vi "adjustDACjob.vi"(10 "sample sn":string[](array[string]), 11 "sample port":refnum<visa-resource-name>[](array[refnum])) -> ()   [LabVIEW 2012]
uses:
  globalstatus.vi
  globalsettings.vi
  globalreport.vi
panel:
  out "min":dbl[](array[numeric])
  out "max":dbl[](array[numeric])
  out "real pool":dbl[][](array[numeric])
  in  "times":dbl
  in  "count":dbl
  out "error":errorcluster[](array[cluster])
  in  "blue amp":dbl[](array[numeric])
  in  "red amp":dbl[](array[numeric])
  in  "isred":bool
  out "image":dbl[](array[numeric])
  out "real":dbl[](array[numeric])
  in  "blue dac":dbl[](array[numeric])
  in  "red dac":dbl[](array[numeric])
  in  "Ring":u16(ring) items=["set DAC", "excite", "read"]
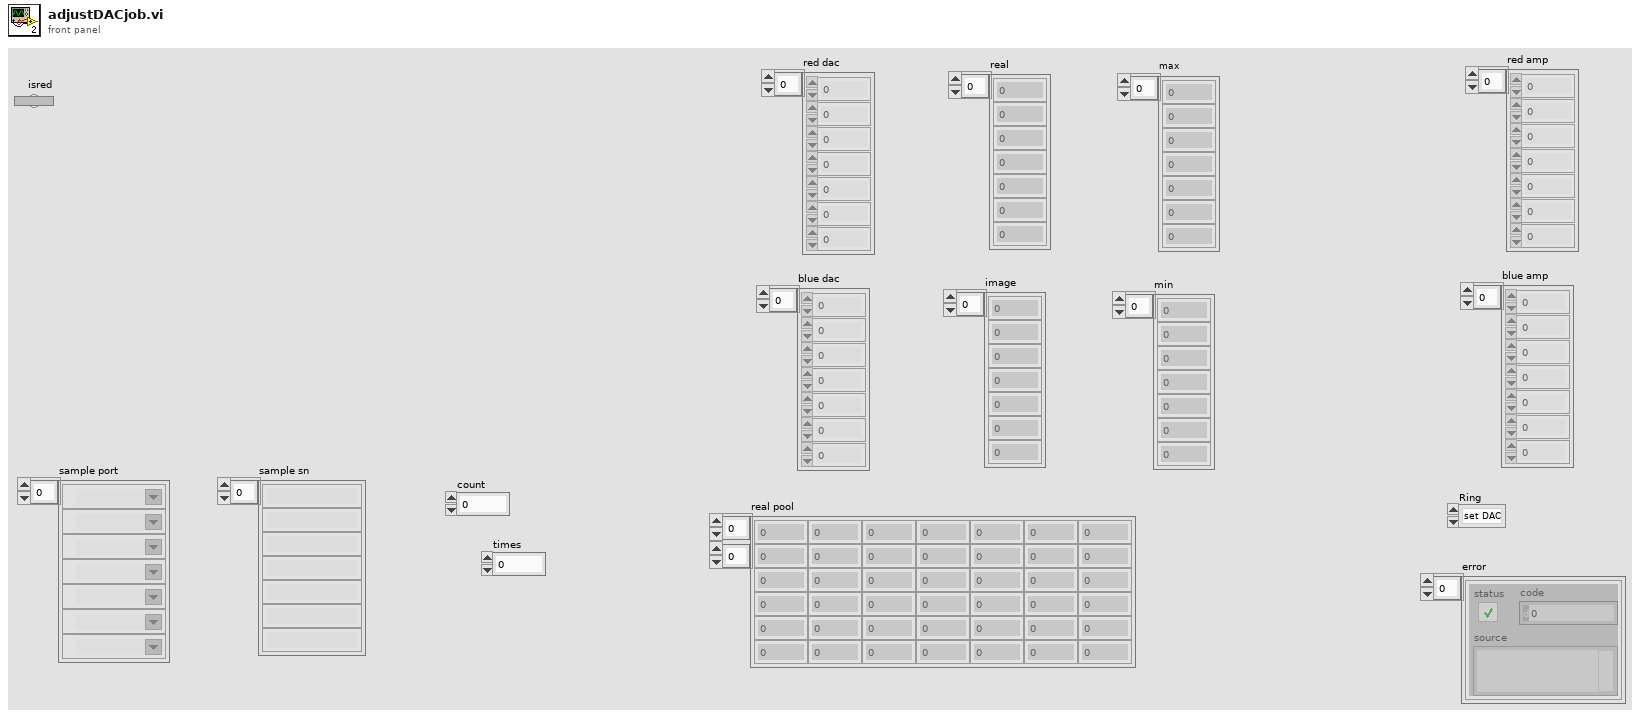
[diagram p1: front panel]
types:
  T1 = cluster{"DAC max":dbl, "DAC min":dbl, "DAC base":dbl, "DAC step":dbl, "Amplitude":dbl, "Tolerance":dbl, "Times":dbl}
  T2 = cluster{"PORT":string, "SN":string, "RED DAC":dbl, "BLUE DAC":dbl, "RED AMP":dbl, "BLUE AMP":dbl, "T0":dbl, "T1":dbl, "T2":dbl, "T3":dbl, "T4":dbl, "T5":dbl, "T6":dbl, "A0":dbl, "A1":dbl, "A2":dbl, "A3":dbl, "B0":dbl, "B1":dbl, "B2":dbl, "C1":dbl, "C0":dbl, "result":string, "error":string}[]
  T3 = cluster{"PORT":string, "SN":string, "RED DAC":dbl, "BLUE DAC":dbl, "RED AMP":dbl, "BLUE AMP":dbl, "T0":dbl, "T1":dbl, "T2":dbl, "T3":dbl, "T4":dbl, "T5":dbl, "T6":dbl, "A0":dbl, "A1":dbl, "A2":dbl, "A3":dbl, "B0":dbl, "B1":dbl, "B2":dbl, "C1":dbl, "C0":dbl, string, string}
  T4 = cluster{"PORT":string, "SN":string, "Numeric":dbl, "Numeric":dbl, "Numeric":dbl, "Numeric":dbl, "T0":dbl, "T1":dbl, "T2":dbl, "T3":dbl, "T4":dbl, "T5":dbl, "T6":dbl, "A0":dbl, "A1":dbl, "A2":dbl, "A3":dbl, "B0":dbl, "B1":dbl, "B2":dbl, "C1":dbl, "C0":dbl, "result":string, "error":string}
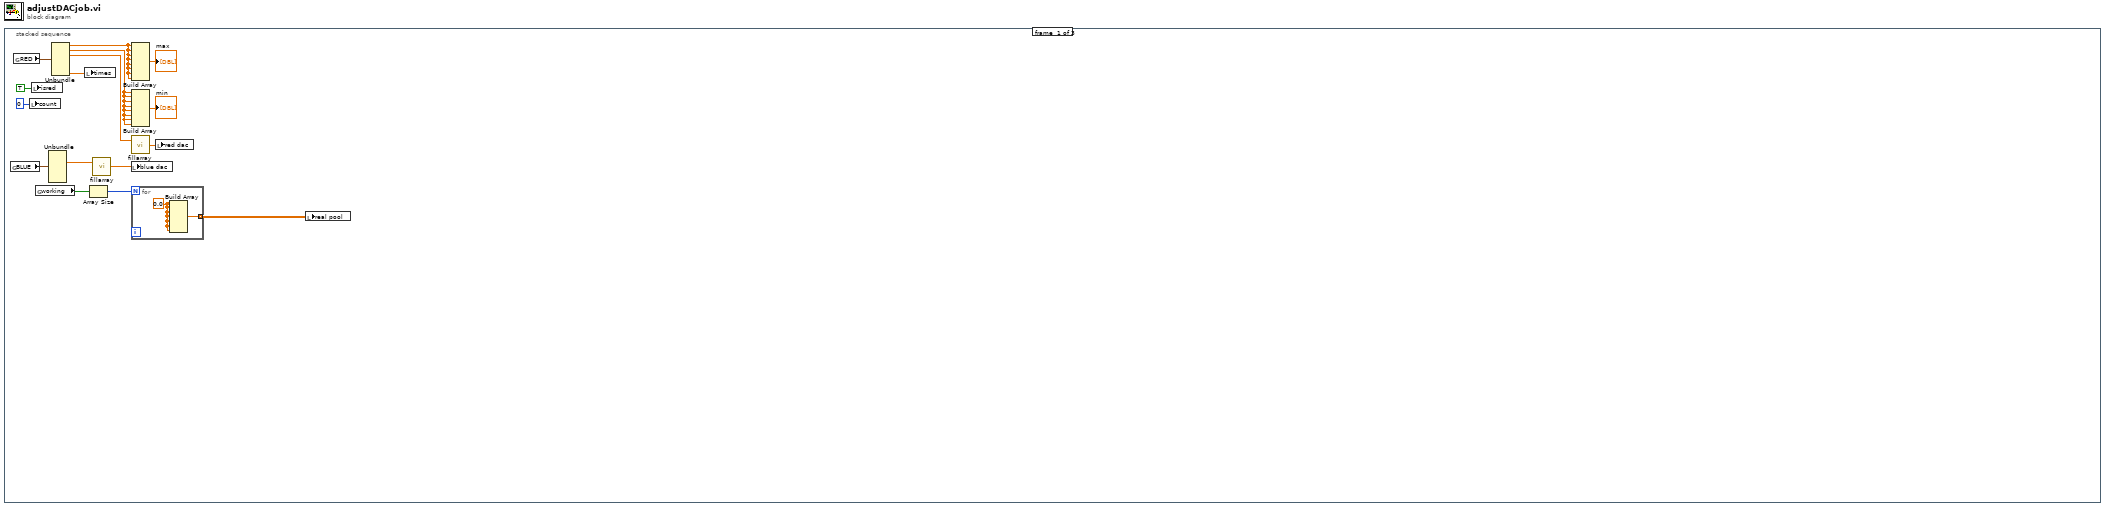
[diagram p0: block diagram]
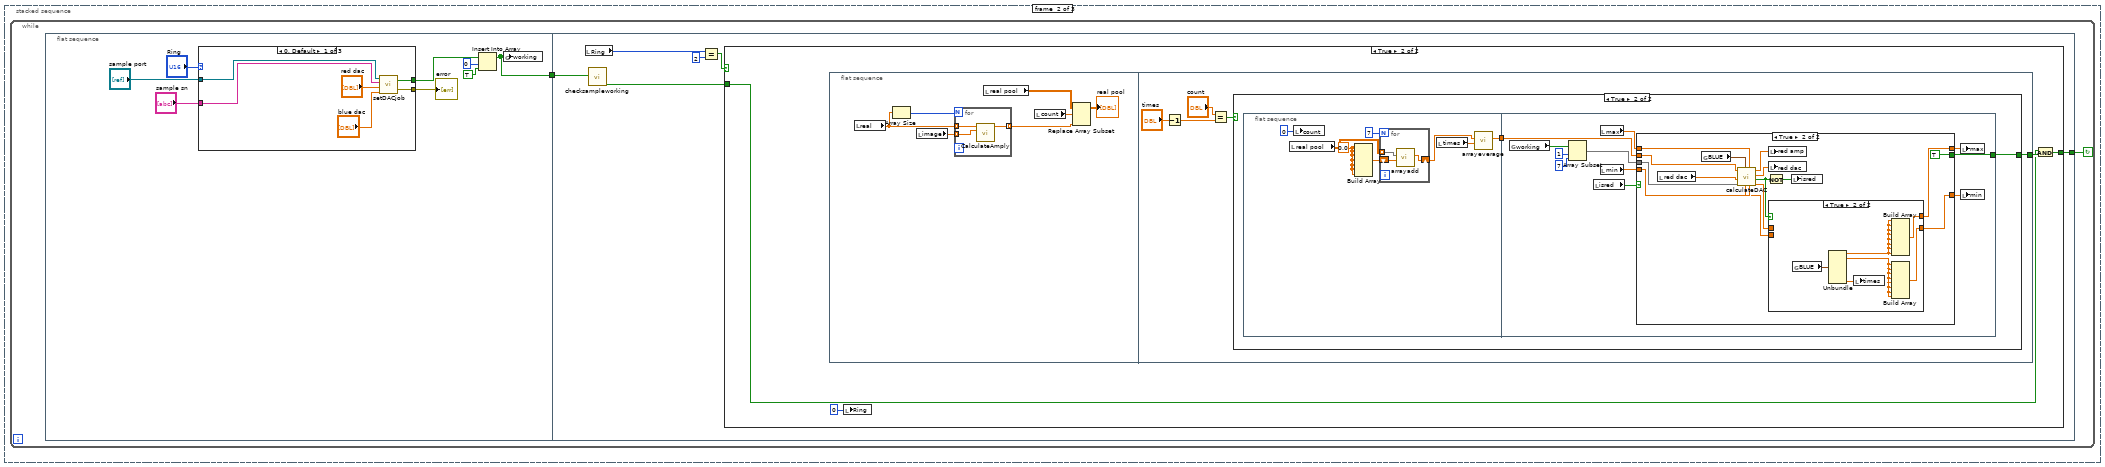
[diagram p2: hidden frame]
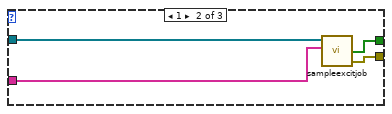
[diagram p3: hidden frame]
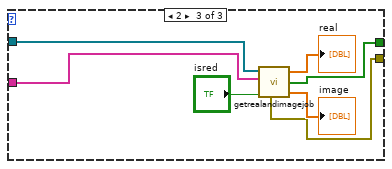
[diagram p4: hidden frame]
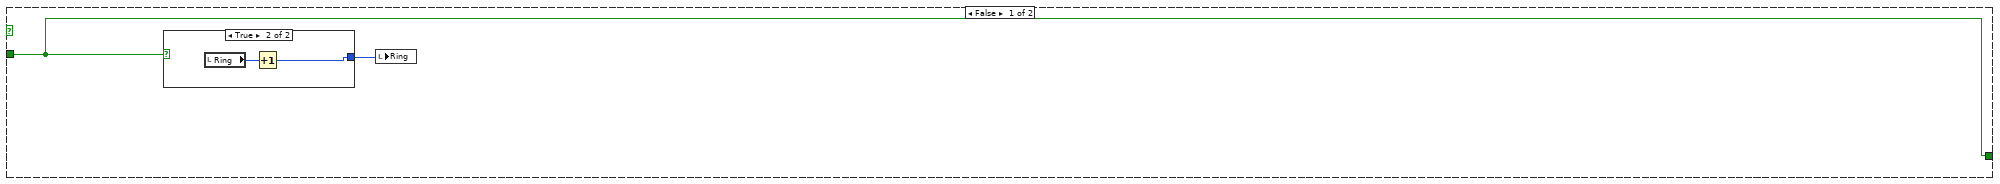
[diagram p5: hidden frame]
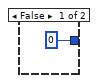
[diagram p6: hidden frame]
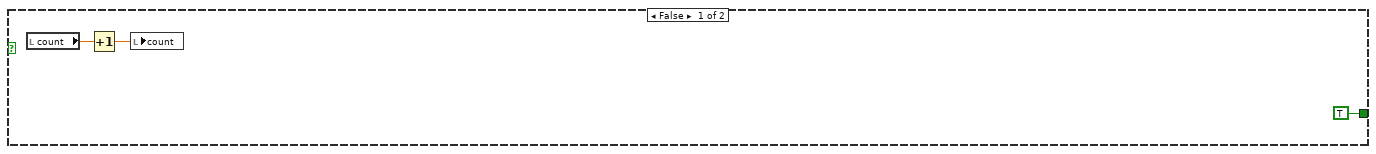
[diagram p7: hidden frame]
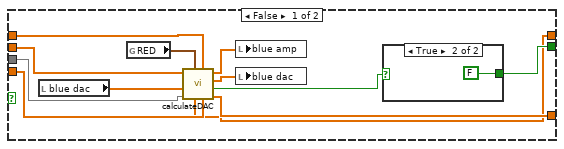
[diagram p8: hidden frame]
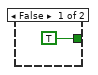
[diagram p9: hidden frame]
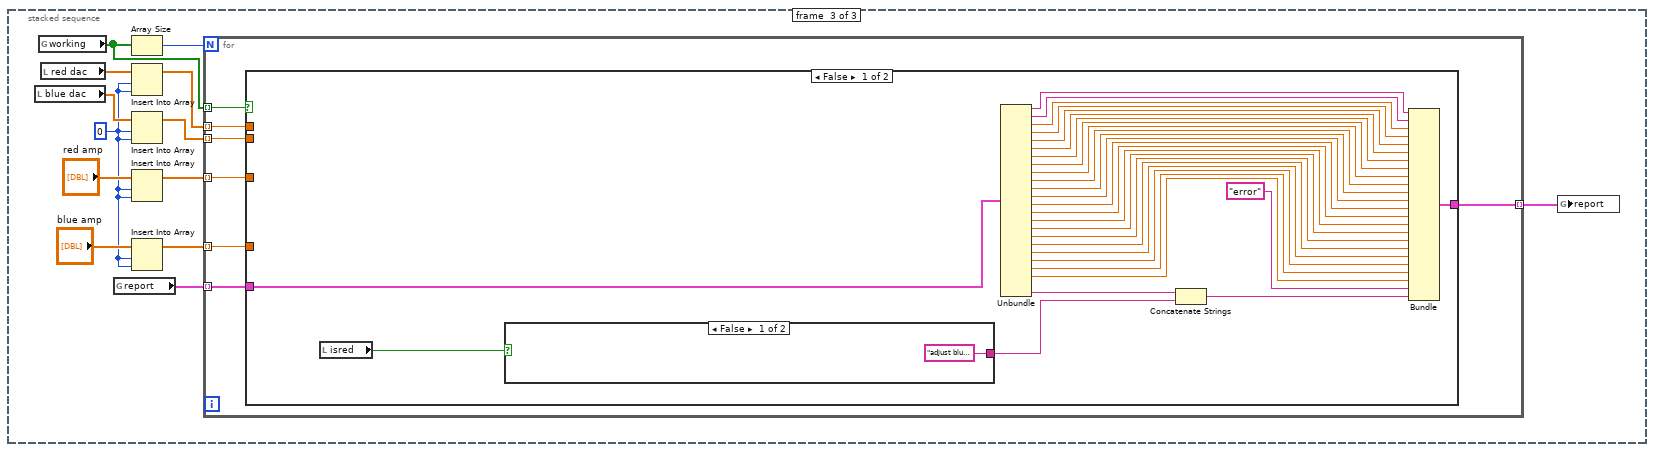
[diagram p11: hidden frame]
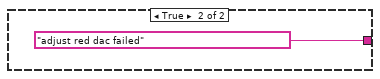
[diagram p12: hidden frame]
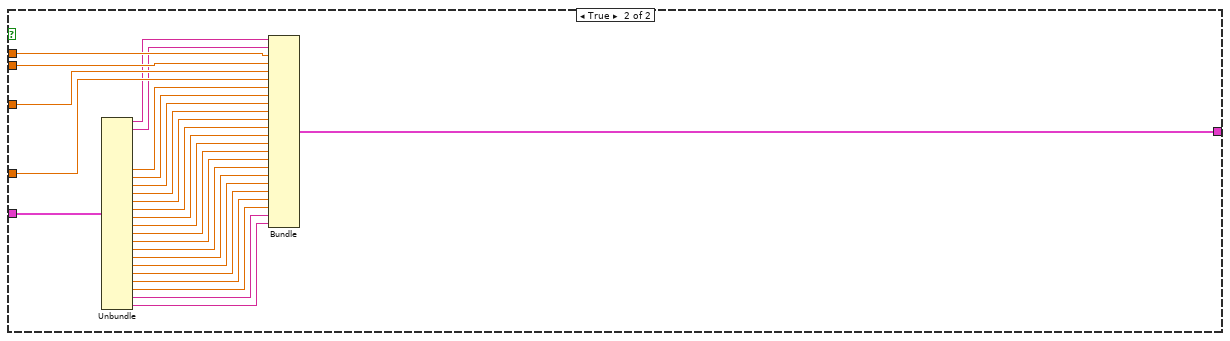
[diagram p13: hidden frame]
diagram:
  n1 = stacked-sequence {
    frame #0 {
      n2 = global read "globalsettings.vi" "BLUE"() -> (w7:T1)
      n3 = global read "globalsettings.vi" "RED"() -> (w8:T1)
      n4 = local write "count"(0) -> ()
      n5 = local write "isred"(TRUE) -> ()
      n6 = global read "globalstatus.vi" "working"() -> (w5:bool[])
      n7 = Unbundle(w7) -> ("DAC base"=w13:dbl)  [unwired: 6 out]
      n8 = Unbundle(w8) -> ("DAC max"=w11:dbl, "DAC min"=w12:dbl, "DAC base"=w14:dbl, "Times"=w6:dbl)  [unwired: 3 out]
      n9 = local write "times"(w6) -> ()
      n10 = Array Size(array=w5) -> (size(s)=w4:i32)
      n11 = call "fillarray.vi"("Numeric"=w13) -> ("Array"=w16:dbl[])  [unwired: 2 in]
      n12 = Build Array(w11, w11, w11, w11, w11, w11, w11, w11) -> (→"max":dbl[])
      n13 = Build Array(w12, w12, w12, w12, w12, w12, w12, w12) -> (→"min":dbl[])
      n14 = call "fillarray.vi"("Numeric"=w14) -> ("Array"=w15:dbl[])  [unwired: 2 in]
      n15 = local write "blue dac"(w16) -> ()
      n16 = for {
        N: w4 -> [_]
        tunnel: [w17] -> w3 mode=indexing
        w18 = 0.0
        n17 = Build Array(w18, w18, w18, w18, w18, w18, w18) -> (w17:dbl[])
      }
      n18 = local write "red dac"(w15) -> ()
      n19 = local write "real pool"(w3) -> ()
    }
    frame #1 {
      n20 = while {
        stop <- w20 continue-if-true
        n21 = flat-sequence {
          tunnel: [w21] -> w19
          tunnel: [w48] -> w20
          tunnel: w19 -> [w46]
          frame #0 {
            n22 = case shown="0, Default" "Ring" {
              tunnel: "sample sn" -> [w32 w37 w43]
              tunnel: "sample port" -> [w31 w38 w42]
              tunnel: [w30 w36 w44] -> w24
              tunnel: [w29 w35 w39] -> w25
              frame 0, Default {
                n23 = call "setDACjob.vi"("blue"="blue dac", "red"="red dac", "sample sn"=w32, "sample port"=w31) -> ("error"=w29:errorcluster[], "Array"=w30:bool[])  [unwired: 2 in]
              }
              frame 1 {
                n24 = call "sampleexcitjob.vi"("sample port"=w38, "sample sn"=w37) -> ("Array"=w36:bool[], "error"=w35:errorcluster[])  [unwired: 5 in]
              }
              frame 2 {
                n25 = call "getrealandimagejob.vi"("sample port"=w42, "sample sn"=w43, "isred"="isred") -> ("error"=w39:errorcluster[], "real"=→"real":dbl[], "Array"=w44:bool[], "image"=→"image":dbl[])  [unwired: 2 in]
              }
            }
            "error" <- w25
            n26 = Insert Into Array(array=w24, index=0, new element=TRUE) -> (w21:bool[])
            n27 = global write "globalstatus.vi" "working"(w21) -> ()
          }
          frame #1 {
            n28 = local read "Ring"() -> (w50:u16)
            n29 = call "checksampleworking.vi"("Array"=w46) -> ("Boolean"=w47:bool)  [unwired: 8 in]
            n30 = Equal?(x=w50, y=2) -> (x = y?=w49:bool)
            n31 = case shown="True" w49 {
              tunnel: [w52 w59] -> w48
              tunnel: w47 -> [w52 w58]
              frame False {
                n32 = case shown="True" w52 {
                  tunnel: [0 w55] -> w53
                  frame False {
                  }
                  frame True {
                    n33 = local read "Ring"() -> (w56:u16)
                    n34 = Increment(x=w56) -> (x+1=w55:u16)
                  }
                }
                n35 = local write "Ring"(w53) -> ()
              }
              frame True {
                n36 = flat-sequence {
                  tunnel: [w75] -> w60
                  frame #0 {
                    n37 = local read "real"() -> (w63:dbl[])
                    n38 = Array Size(array=w63) -> (size(s)=w64:i32)
                    n39 = local read "image"() -> (w62:dbl[])
                    n40 = for {
                      N: w64 -> [_]
                      tunnel: w63 -> [w70] mode=indexing
                      tunnel: w62 -> [w69] mode=indexing
                      tunnel: [w68] -> w61 mode=indexing
                      n41 = call "CalculateAmply.vi"("image"=w69, "real"=w70) -> ("amply"=w68:dbl)  [unwired: 9 in]
                    }
                    n42 = local read "real pool"() -> (w67:dbl[][])
                    n43 = local read "count"() -> (w65:dbl)
                    n44 = Replace Array Subset(array=w67, new element=w61, index (row)=w65) -> (→"real pool":dbl[][])  [unwired: 1 in]
                  }
                  frame #1 {
                    n45 = Decrement(x="times") -> (x-1=w71:dbl)
                    n46 = Equal?(x="count", y=w71) -> (x = y?=w74:bool)
                    n47 = case shown="True" w74 {
                      tunnel: [TRUE w80] -> w75
                      frame False {
                        n48 = local read "count"() -> (w77:dbl)
                        n49 = Increment(x=w77) -> (x+1=w76:dbl)
                        n50 = local write "count"(w76) -> ()
                      }
                      frame True {
                        n51 = flat-sequence {
                          tunnel: [w83] -> w79
                          tunnel: [w101] -> w80
                          tunnel: w79 -> [w100]
                          frame #0 {
                            w85 = 0.0
                            n52 = local read "real pool"() -> (w88:dbl[][])
                            n53 = local write "count"(0) -> ()
                            n54 = Build Array(w85, w85, w85, w85, w85, w85, w85) -> (w86:dbl[])
                            n55 = for {
                              N: 7 -> [_]
                              tunnel: w88 -> [w91] mode=indexing
                              shift-right: [w90] -> w84
                              shift-left: w86 -> [w89]
                              n56 = call "arrayadd.vi"("b"=w89, "a"=w91) -> ("c"=w90:dbl[])  [unwired: 9 in]
                            }
                            n57 = local read "times"() -> (w82:dbl)
                            n58 = call "arrayeverage.vi"("divider"=w82, "in"=w84) -> ("out"=w83:dbl[])  [unwired: 9 in]
                          }
                          frame #1 {
                            n59 = global read "globalstatus.vi" "working"() -> (w95:bool[])
                            n60 = Array Subset(array=w95, index=1, length=7) -> (w92:bool[])
                            n61 = local read "isred"() -> (w102:bool)
                            n62 = local read "max"() -> (w99:dbl[])
                            n63 = local read "min"() -> (w98:dbl[])
                            n64 = case shown="True" w102 {
                              tunnel: w100 -> [w114 w130]
                              tunnel: [w110 TRUE] -> w101
                              tunnel: w92 -> [w109 w126]
                              tunnel: w99 -> [w107 w124]
                              tunnel: w98 -> [w106 w123]
                              tunnel: [w104 w118] -> w97
                              tunnel: [w105 w121] -> w96
                              frame False {
                                n65 = local read "blue dac"() -> (w113:dbl[])
                                n66 = global read "globalsettings.vi" "RED"() -> (w103:T1)
                                n67 = call "calculateDAC.vi"("min"=w106, "max"=w107, "settings"=w103, "working"=w109, "old DAC"=w113, "real"=w114) -> ("new min"=w105:dbl[], "isok"=w111:bool, "new DAC"=w112:dbl[], "amplitude"=w108:dbl[], "new max"=w104:dbl[])  [unwired: 1 in]
                                n68 = local write "blue amp"(w108) -> ()
                                n69 = local write "blue dac"(w112) -> ()
                                n70 = case shown="True" w111 {
                                tunnel: [TRUE FALSE] -> w110
                                frame False {
                                }
                                frame True {
                                }
                                }
                              }
                              frame True {
                                n71 = local read "red dac"() -> (w131:dbl[])
                                n72 = global read "globalsettings.vi" "BLUE"() -> (w117:T1)
                                n73 = call "calculateDAC.vi"("min"=w123, "max"=w124, "settings"=w117, "working"=w126, "old DAC"=w131, "real"=w130) -> ("new min"=w120:dbl[], "isok"=w122:bool, "new DAC"=w129:dbl[], "amplitude"=w125:dbl[], "new max"=w119:dbl[])  [unwired: 1 in]
                                n74 = Not(x=w122) -> (.not. x?=w128:bool)
                                n75 = local write "red amp"(w125) -> ()
                                n76 = local write "red dac"(w129) -> ()
                                n77 = case shown="True" w122 {
                                tunnel: w120 -> [w133 _]
                                tunnel: [w133 w136] -> w121
                                tunnel: w119 -> [w132 _]
                                tunnel: [w132 w137] -> w118
                                frame False {
                                }
                                frame True {
                                n78 = global read "globalsettings.vi" "BLUE"() -> (w135:T1)
                                n79 = Unbundle(w135) -> ("DAC max"=w138:dbl, "DAC min"=w139:dbl, "Times"=w134:dbl)  [unwired: 4 out]
                                n80 = local write "times"(w134) -> ()
                                n81 = Build Array(w138, w138, w138, w138, w138, w138, w138, w138) -> (w137:dbl[])
                                n82 = Build Array(w139, w139, w139, w139, w139, w139, w139, w139) -> (w136:dbl[])
                                }
                                }
                                n83 = local write "isred"(w128) -> ()
                              }
                            }
                            n84 = local write "max"(w97) -> ()
                            n85 = local write "min"(w96) -> ()
                          }
                        }
                      }
                    }
                  }
                }
                n86 = local write "Ring"(0) -> ()
                n87 = And(x=w58, y=w60) -> (x .and. y?=w59:bool)
              }
            }
          }
        }
      }
    }
    frame #2 {
      w140 = 0
      n88 = local read "blue dac"() -> (w148:dbl[])
      n89 = global read "globalstatus.vi" "working"() -> (w141:bool[])
      n90 = local read "red dac"() -> (w149:dbl[])
      n91 = global read "globalreport.vi" "report"() -> (w151:T2)
      n92 = Array Size(array=w141) -> (size(s)=w152:i32)
      n93 = Insert Into Array(array=w149, index=w140, new element=w140) -> (w147:dbl[])
      n94 = Insert Into Array(array=w148, index=w140, new element=w140) -> (w146:dbl[])
      n95 = Insert Into Array(array="red amp", index=w140, new element=w140) -> (w142:dbl[])
      n96 = Insert Into Array(array="blue amp", index=w140, new element=w140) -> (w143:dbl[])
      n97 = for {
        N: w152 -> [_]
        tunnel: w141 -> [w153] mode=indexing
        tunnel: w151 -> [w159] mode=indexing
        tunnel: [w158] -> w150 mode=indexing
        tunnel: w142 -> [w157] mode=indexing
        tunnel: w143 -> [w156] mode=indexing
        tunnel: w147 -> [w155] mode=indexing
        tunnel: w146 -> [w154] mode=indexing
        n98 = case shown="False" w153 {
          tunnel: w159 -> [w188 w216]
          tunnel: [w163 w191] -> w158
          tunnel: w157 -> [_ w196]
          tunnel: w156 -> [_ w197]
          tunnel: w155 -> [_ w195]
          tunnel: w154 -> [_ w194]
          frame False {
            n99 = local read "isred"() -> (w164:bool)
            n100 = case shown="False" w164 {
              tunnel: ["adjust blue dac failed" "adjust red dac failed"] -> w161
              frame False {
              }
              frame True {
              }
            }
            n101 = Unbundle(w188) -> ("PORT"=w187:string, "SN"=w186:string, "RED DAC"=w185:dbl, "BLUE DAC"=w184:dbl, "RED AMP"=w183:dbl, "BLUE AMP"=w182:dbl, "T0"=w181:dbl, "T1"=w180:dbl, "T2"=w179:dbl, "T3"=w178:dbl, "T4"=w177:dbl, "T5"=w176:dbl, "T6"=w175:dbl, "A0"=w174:dbl, "A1"=w173:dbl, "A2"=w172:dbl, "A3"=w171:dbl, "B0"=w170:dbl, "B1"=w169:dbl, "B2"=w168:dbl, "C1"=w167:dbl, "C0"=w166:dbl, "error"=w162:string)  [unwired: 1 out]
            n102 = Concatenate Strings(w162, w161) -> (w160:string)
            n103 = Bundle("PORT"=w187, "SN"=w186, "RED DAC"=w185, "BLUE DAC"=w184, "RED AMP"=w183, "BLUE AMP"=w182, "T0"=w181, "T1"=w180, "T2"=w179, "T3"=w178, "T4"=w177, "T5"=w176, "T6"=w175, "A0"=w174, "A1"=w173, "A2"=w172, "A3"=w171, "B0"=w170, "B1"=w169, "B2"=w168, "C1"=w167, "C0"=w166, "error", w160) -> (w163:T3)  [unwired: 1 in]
          }
          frame True {
            n104 = Unbundle(w216) -> ("PORT"=w192:string, "SN"=w193:string, "T0"=w198:dbl, "T1"=w199:dbl, "T2"=w200:dbl, "T3"=w201:dbl, "T4"=w202:dbl, "T5"=w203:dbl, "T6"=w204:dbl, "A0"=w205:dbl, "A1"=w206:dbl, "A2"=w207:dbl, "A3"=w208:dbl, "B0"=w209:dbl, "B1"=w210:dbl, "B2"=w211:dbl, "C1"=w212:dbl, "C0"=w213:dbl, "result"=w214:string, "error"=w215:string)  [unwired: 4 out]
            n105 = Bundle("PORT"=w192, "SN"=w193, "Numeric"=w195, "Numeric"=w194, "Numeric"=w196, "Numeric"=w197, "T0"=w198, "T1"=w199, "T2"=w200, "T3"=w201, "T4"=w202, "T5"=w203, "T6"=w204, "A0"=w205, "A1"=w206, "A2"=w207, "A3"=w208, "B0"=w209, "B1"=w210, "B2"=w211, "C1"=w212, "C0"=w213, "result"=w214, "error"=w215) -> (w191:T4)  [unwired: 1 in]
          }
        }
      }
      n106 = global write "globalreport.vi" "report"(w150) -> ()
    }
  }
